vi "ukol 3.vi"() -> ()   [LabVIEW 2023]
uses:
  <vilib>/addons/Digital Filter Design/Process.llb/DFD Filtering (Wfm).vi
  <vilib>/measure/maspectr.llb/FFT Spectrum (Mag-Phase) for 1 Chan.vi
  <vilib>/addons/Digital Filter Design/NI_DigFilterLicensed.lvlib
  <vilib>/measure/NI_MAPro.lvlib
  <vilib>/measure/NI_MABase.lvlib
  <vilib>/Analysis/NI_AALPro.lvlib
panel:
  out "XY Graph 6":cluster{dbl[], dbl[]}(graph)
  out "XY Graph 5":cluster{dbl[], dbl[]}(graph)
  out "XY Graph 4":cluster{dbl[], dbl[]}(graph)
  out "XY Graph 3":cluster{dbl[], dbl[]}(graph)
  out "XY Graph 2":cluster{dbl[], dbl[]}(graph)
  out "XY Graph":cluster{dbl[], dbl[]}(graph)
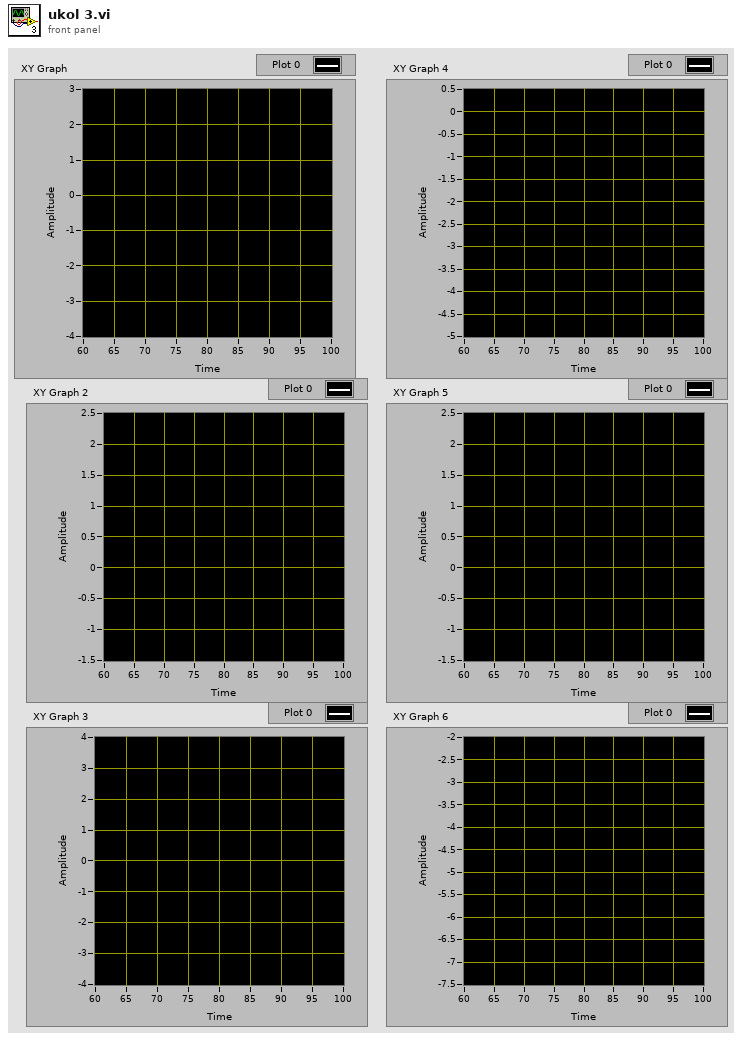
[diagram p1: front panel]
types:
  T1 = cluster{"dB On (F)":bool, "unwrap phase (F)":bool, "convert to degree (F)":bool}
  T2 = typedef "NI_DigFilterLicensed.lvlib/DFD Filter Obj.ctl" = cluster{"mSRate_Fs":dbl, "mSRate_Version":string, "mSRate_Comments":string, "mSRate_OrgCoef":T3, "mSRate_CurCoef":T3, "mSRate_Quantized?":bool, "mSRate_QCoef":T3, "mSRate_QSettings":T5[], "mSRate_Order":i32, "mSRate_Scaling":cluster{"mSRate_ScaleByPowerOf2?":bool, "mSRate_ScaleType":T7}}
  T3 = typedef "NI_DigFilterLicensed.lvlib/DFD Filter Coef.ctl" = cluster{"type":T4, "gain":dbl, "coef a (k)":dbl[], "coef b (v)":dbl[]}
  T4 = typedef "NI_DigFilterLicensed.lvlib/DFD Filter Structure Type Selector.ctl" = enum16{"Undefined", "FIR Direct Form", "FIR Direct Form Transposed", "FIR Symmetric", "FIR Antisymmetric", "IIR Direct Form I", "IIR Direct Form I Transposed", "IIR Direct Form II", "IIR Direct Form II Transposed", "IIR Cascaded Second Order Sections Form I", "IIR Cascaded Second Order Sections Form I Transposed", "IIR Cascaded Second Order Sections Form II", "IIR Cascaded Second Order Sections Form II Transposed", "Lattice Allpass (basic sections)", "Lattice Allpass (one multiplier sections)", "Lattice Allpass (normalized sections)", "Lattice AR (basic sections)", "Lattice AR (one multiplier sections)", "Lattice AR (normalized sections)", "Lattice MA (minimum phase)", "Lattice MA (maximum phase)", "Lattice ARMA (basic sections)", "Lattice ARMA (one multiplier sections)", "Lattice ARMA (normalized sections)"}
  T5 = typedef "NI_DigFilterLicensed.lvlib/dfd_Internal Quantization Settings.ctl" = cluster{"source":T6, "wl":i16, "iwl":i16, "overflow mode":enum16{"Saturation", "Wrap"}, "rounding mode":enum16{"Nearest", "Truncation"}, "signed?":bool}
  T6 = typedef "NI_DigFilterLicensed.lvlib/dfd_Internal Quantization Srcs.ctl" = u16
  T7 = typedef "NI_DigFilterLicensed.lvlib/DFD Coef Norm Type.ctl" = enum16{"No Norm", "Time Domain 1-Norm", "Time Domain 2-Norm", "Time Domain Inf-Norm"}
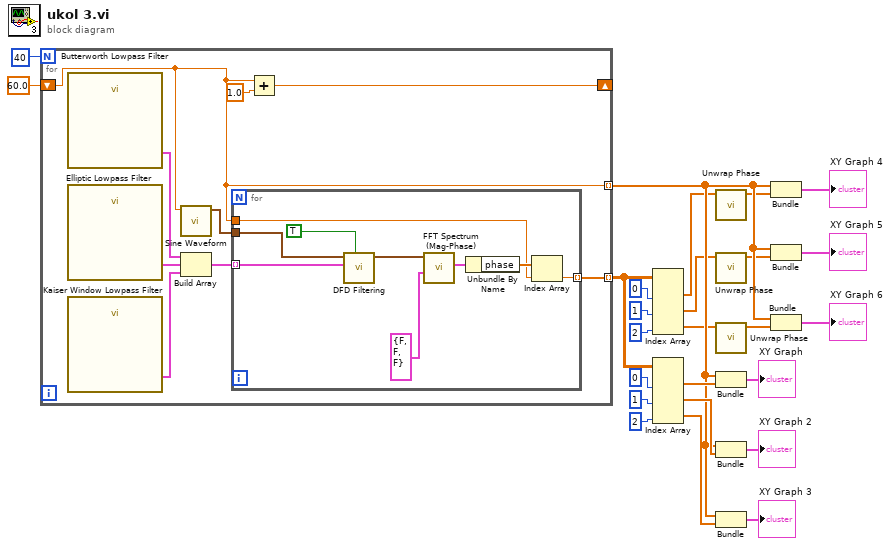
[diagram p0: block diagram]
diagram:
  n1 = for {
    N: 40 -> [_]
    shift-right: [w32] -> _
    shift-left: 60.0 -> [w27]
    tunnel: [w26] -> w10 mode=indexing
    tunnel: [w27] -> w11 mode=indexing
    n2 = call "Butterworth Lowpass Filter"() -> ("filter out"=w29:T2)  [unwired: 10 in, 1 out]
    n3 = call "Elliptic Lowpass Filter"() -> ("filter out"=w30:T2)  [unwired: 10 in, 1 out]
    n4 = call "Kaiser Window Lowpass Filter"() -> ("filter out"=w31:T2)  [unwired: 10 in, 1 out]
    n5 = call <vilib>:"Sine Waveform.vi"("frequency"=w27) -> ("signal out"=w33:waveform(dbl))  [unwired: 9 in, 1 out]
    n6 = Build Array(w29, w30, w31) -> (w28:T2[])
    n7 = for {
      tunnel: w33 -> [w41]
      tunnel: w27 -> [w38]
      tunnel: [w37] -> w26 mode=indexing
      tunnel: w28 -> [w36] mode=indexing
      n8 = call-poly <vilib>:"DFD Filtering.vi"("init? (F)"=TRUE, "filter"=w36, "signal in"=w41) -> ("signal out"=w35:waveform(dbl))  [unwired: 7 in, 1 out]
      n9 = call-poly <vilib>:"FFT Spectrum (Mag-Phase).vi"("view"=T1 {"dB On (F)"=FALSE, "unwrap phase (F)"=FALSE, "convert to degree (F)"=FALSE}, "time signal"=w35) -> ("phase"=w40:cluster{"f0":dbl, "df":dbl, "phase":dbl[]})  [unwired: 5 in, 4 out]
      n10 = Unbundle By Name(w40) -> ("phase"=w39:dbl[])
      n11 = Index Array(array=w39, index=w38) -> (element=w37:dbl)
    }
    n12 = Add(x=w27, y=1.0) -> (x+y=w32:dbl)
  }
  n13 = Index Array(array=w10, index (col) #1=0 ("index"), index (col) #2=1 ("index"), index (col) #3=2 ("index")) -> (element #1=w9:dbl[], element #2=w7:dbl[], element #3=w5:dbl[])  [unwired: 3 in]
  n14 = Index Array(array=w10, index (col) #1=0 ("index"), index (col) #2=1 ("index"), index (col) #3=2 ("index")) -> (element #1=w23:dbl[], element #2=w21:dbl[], element #3=w20:dbl[])  [unwired: 3 in]
  n15 = call <vilib>:"Unwrap Phase.vi"("Phase"=w9) -> ("Unwrapped Phase"=w8:dbl[])  [unwired: 9 in, 1 out]
  n16 = call <vilib>:"Unwrap Phase.vi"("Phase"=w7) -> ("Unwrapped Phase"=w6:dbl[])  [unwired: 9 in, 1 out]
  n17 = call <vilib>:"Unwrap Phase.vi"("Phase"=w5) -> ("Unwrapped Phase"=w4:dbl[])  [unwired: 9 in, 1 out]
  n18 = Bundle(w11, w23) -> (→"XY Graph":cluster{dbl[], dbl[]})  [unwired: 1 in]
  n19 = Bundle(w11, w21) -> (→"XY Graph 2":cluster{dbl[], dbl[]})  [unwired: 1 in]
  n20 = Bundle(w11, w20) -> (→"XY Graph 3":cluster{dbl[], dbl[]})  [unwired: 1 in]
  n21 = Bundle(w11, "Unwrapped Phase"=w8) -> (→"XY Graph 4":cluster{dbl[], "Unwrapped Phase":dbl[]})  [unwired: 1 in]
  n22 = Bundle(w11, "Unwrapped Phase"=w6) -> (→"XY Graph 5":cluster{dbl[], "Unwrapped Phase":dbl[]})  [unwired: 1 in]
  n23 = Bundle(w11, "Unwrapped Phase"=w4) -> (→"XY Graph 6":cluster{dbl[], "Unwrapped Phase":dbl[]})  [unwired: 1 in]
